vi "Cal Sets  Copy.vi"(8 "error in (no error)":errorcluster {"code" format="%.0x"}, 9 "NewCalSet":string, 10 "OldCalSet":string, 11 "instrument handle":refnum<k15>) -> (0 "error out":errorcluster {"code" format="%.0x"}, 3 "instrument handle out":refnum<k15>)   [LabVIEW 2014, in "Agilent NA.lvlib"]
doc: "Copy the specified Cal Set to a new cal set."
uses:
  Agilent NA.lvlib
  AgNA.dll
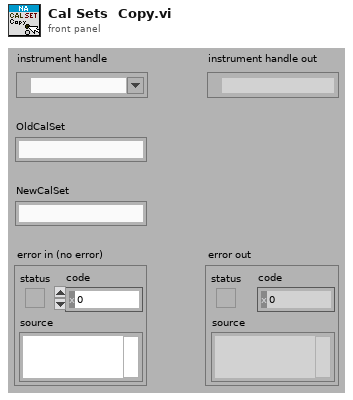
[diagram p1: front panel]
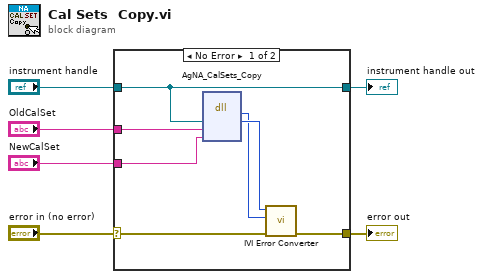
[diagram p0: block diagram]
diagram:
  n1 = case shown="No Error" "error in (no error)" {
    selector: "error in (no error)" -> [w11 w15]
    tunnel: [w10 w15] -> w6
    tunnel: "OldCalSet" -> [w9 _]
    tunnel: "NewCalSet" -> [w8 _]
    tunnel: [w7 w14] -> w2
    tunnel: "instrument handle" -> [w7 w14]
    frame No Error {
      n2 = dll-call lib="AgNA**.dll" fn="AgNA_CalSets_Copy"("Vi"=w7, "OldCalSet"=w9, "NewCalSet"=w8) -> (w12:i32, "Vi"=w13:u32)  [unwired: 5 in, 2 out]
      n3 = call "IVI Error Converter.vi"("error in (no error)"=w11, "IVI error code (0)"=w12, "instrument handle"=w13) -> ("error out"=w10:errorcluster)  [unwired: 7 in, 1 out]
    }
    frame Error {
    }
  }
  "error out" <- w6
  "instrument handle out" <- w2
